vi "ingest.avro_stream.vi"(8 "error in":errorcluster, 11 "Client in":refnum<class "Client.lvclass">) -> (0 "error out":errorcluster, 3 "Client out":refnum<class "Client.lvclass">)   [LabVIEW 2020, in "Client.lvclass"]
doc: "Ingests a Nominal Avro-stream file into an existing dataset."
uses:
  Client.lvclass
  Client.lvclass/Client.ctl
  client.lvlib
panel:
  out "out_job out":i32
  in  "file_path":string
  in  "dataset_rid":string
  in  "out_job":i32
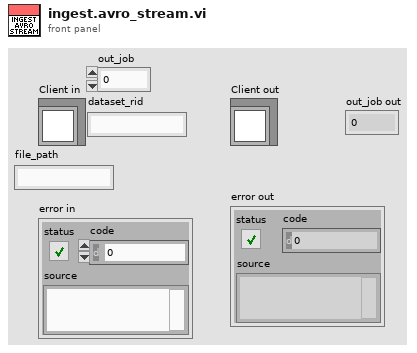
[diagram p1: front panel]
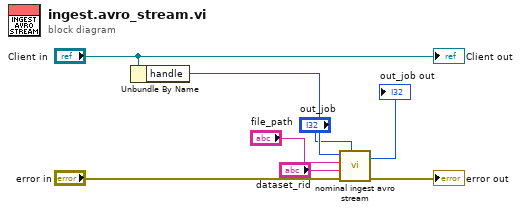
[diagram p0: block diagram]
diagram:
  n1 = Unbundle By Name("Client in") -> ("handle"=w6:i32)
  n2 = call "nominal ingest avro stream.vi"("out_job"="out_job", "error in (no error)"="error in", "dataset_rid"="dataset_rid", "file_path"="file_path", "client"=w6) -> ("error out"=→"error out":errorcluster, "out_job out"=→"out_job out":i32)  [unwired: 4 in, 1 out]
  "Client out" <- "Client in"
